vi "read eip channels.vi"(8 "error in (no error)":errorcluster, 11 "EthernetIP configuration in":refnum<class "EthernetIP configuration.lvclass">) -> (0 "error out":errorcluster, 2 "channels":refnum<class "EthernetIP Channel.lvclass">[](array[class]), 3 "EthernetIP configuration out":refnum<class "EthernetIP configuration.lvclass">)   [LabVIEW 2013, in "EthernetIP configuration.lvclass"]
uses:
  EthernetIP configuration.lvclass
  channel/EthernetIP Channel.lvclass
  EthernetIP configuration.lvclass/EthernetIP configuration.ctl
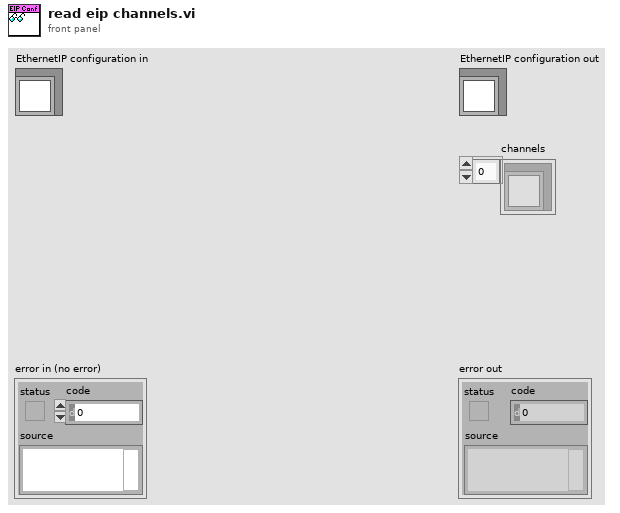
[diagram p1: front panel]
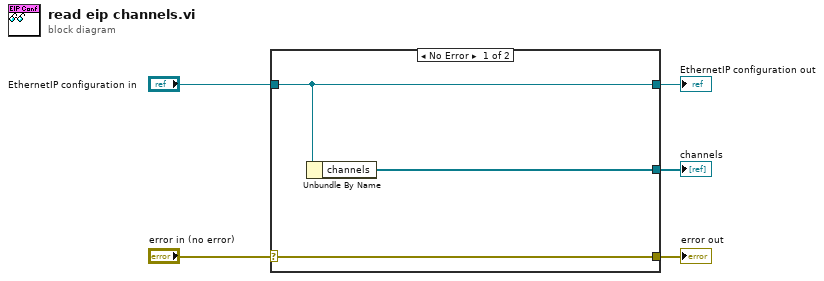
[diagram p0: block diagram]
diagram:
  n1 = case shown="No Error" "error in (no error)" {
    selector: "error in (no error)" -> [w8 w9]
    tunnel: [w8 w9] -> w4
    tunnel: [w7 w10] -> w2
    tunnel: "EthernetIP configuration in" -> [w7 w10]
    tunnel: [w6 _] -> w1
    frame No Error {
      n2 = Unbundle By Name(w7) -> ("channels"=w6:refnum<class "EthernetIP Channel.lvclass">[])
    }
    frame Error {
    }
  }
  "error out" <- w4
  "EthernetIP configuration out" <- w2
  "channels" <- w1
